vi "Arduino Interfacing VI.vi"(2 "error in (no error)":errorcluster, 3 "y Stepper value":u8, 4 "Data to Write":T1, 5 "AE Mode":T2) -> (0 "error out":errorcluster, 1 "Arduino Data":T3)   [LabVIEW 2018]
uses:
  Arduino_Interfacing.ctl
  I2C_MASTER_WRITE_NEW Type Def.ctl
  <vilib>/Studica/Studica Toolkit/Background/I2C Channel.ctl
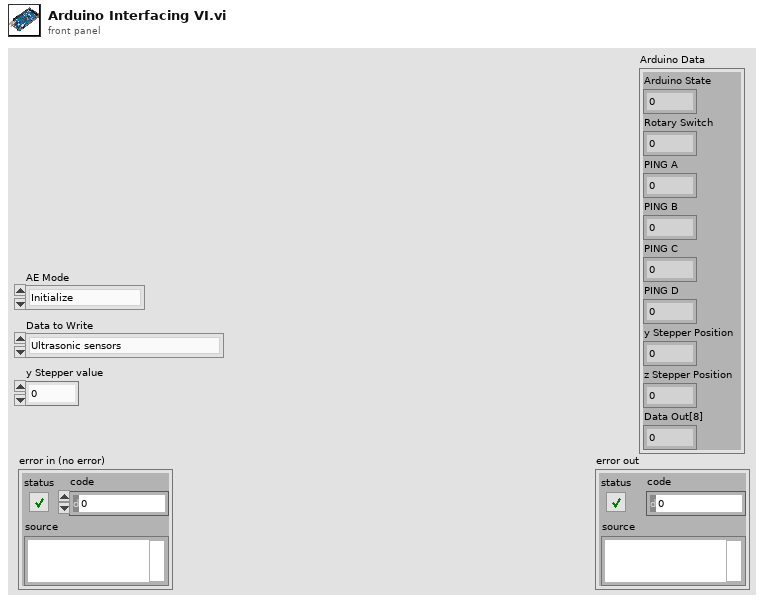
[diagram p1: front panel]
types:
  T1 = typedef "I2C_MASTER_WRITE_NEW Type Def.ctl" = enum16{"Ultrasonic sensors", "Stepper origin", "zStepper 13.3k", "zStepper 13k", "zStepper 12k", "zStepper 11k", "zStepper 10k", "zStepper 9k", "zStepper 8k", "zStepper 7k", "zStepper 6k", "zStepper 5k", "zStepper 4k", "zStepper 3k", "zStepper 2k", "zStepper 1k", "zStepper 900", "zStepper 800", "zStepper 700", "zStepper 600", "zStepper 500", "zStepper 400", "zStepper 300", "zStepper 200", "zStepper 100", "zStepper 0", "yStepper control", "Open Claw", "Close Claw", "Soft Reset"}
  T2 = typedef "Arduino_Interfacing.ctl" = enum16{"Initialize", "Write to Arduino", "Read From Arduino"}
  T3 = cluster{"Arduino State":u8, "Rotary Switch":u8, "PING A":u8, "PING B":u8, "PING C":u8, "PING D":u8, "y Stepper Position":u8, "z Stepper Position":u8, "Data Out[8]":u8}
  T4 = typedef "I2C Channel.ctl" = enum16{"Not Connected", "A", "B"}
  T5 = cluster{"I2C Channel":T4, "FPGA VI Reference Out":refnum<k20>}
  T6 = cluster{"Data Out[0]":u8, "Data Out[1]":u8, "Data Out[2]":u8, "Data Out[3]":u8, "Data Out[4]":u8, "Data Out[5]":u8, "Data Out[6]":u8, "Data Out[7]":u8, "Data Out[8]":u8}
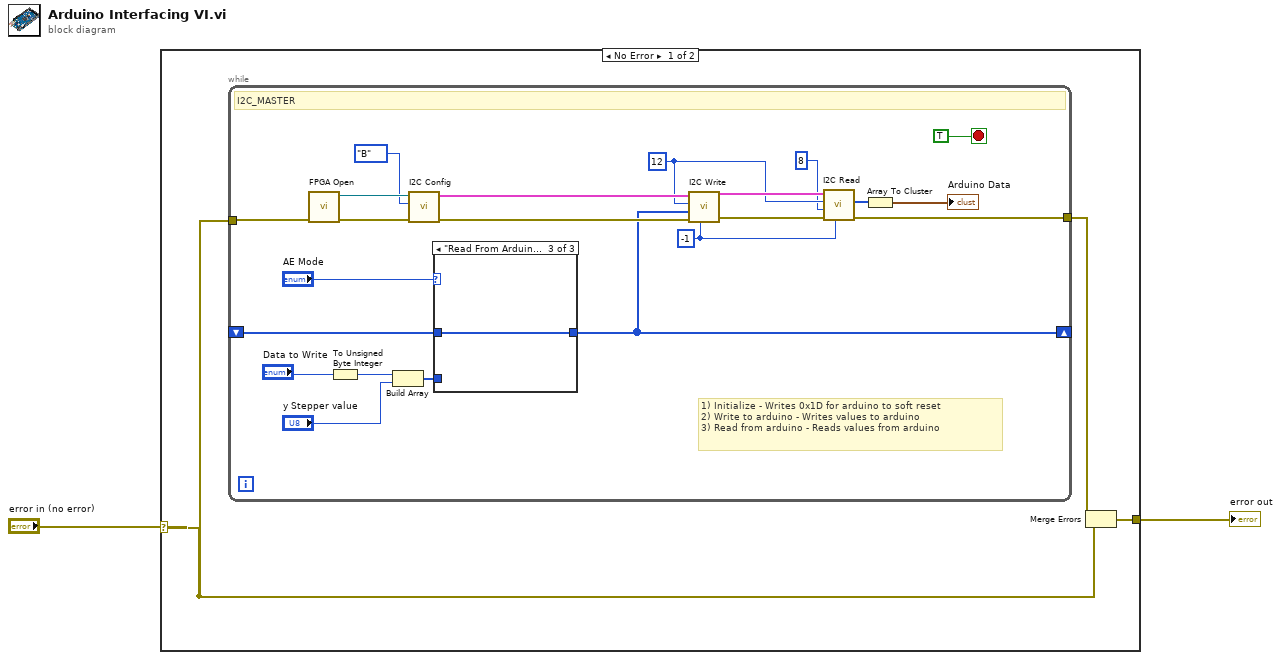
[diagram p0: block diagram]
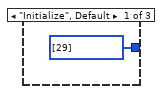
[diagram p2: hidden frame]
diagram:
  n1 = case shown="No Error" "error in (no error)" {
    selector: "error in (no error)" -> [w4 w31]
    tunnel: [w5 w31] -> w1
    frame No Error {
      n2 = while {
        tunnel: w4 -> [w21]
        shift-right: [w9] -> _
        shift-left: _ -> [w8]
        tunnel: [w13] -> w3
        stop <- TRUE ("stop") stop-if-true
        w16 = -1 ("Timeout ms (1000)")
        w15 = u8 12 ("Slave Address (7-bit)")
        # "1) Initialize - Writes 0x1D for arduino to soft reset\n2) Write to arduino - Writes values to arduino\n3) Read from arduino - Reads values from arduino"
        # "I2C_MASTER"
        n3 = call <vilib>:"FPGA Open.vi"("error in (no error)"=w21) -> ("error out"=w25:errorcluster, "FPGA Reference Out"=w26:refnum<k20>)  [unwired: 9 in]
        n4 = To Unsigned Byte Integer(number="Data to Write") -> (unsigned 8bit integer=w20:u8)
        n5 = Build Array(w20, "y Stepper value") -> (w10:u8[])
        n6 = call <vilib>:"I2C Config.vi"("error in (no error)"=w25, "I2C Channel"=I2C_Channel."B", "FPGA Reference"=w26) -> ("error out"=w22:errorcluster, "I2C Ref Out"=w23:T5)  [unwired: 7 in]
        n7 = case shown="\"Read From Arduino\"" "AE Mode" {
          tunnel: [u8[] [29] ("Data to Write") w29 w30] -> w9
          tunnel: w10 -> [_ w29 _]
          tunnel: w8 -> [_ _ w30]
          frame "Initialize", Default {
          }
          frame "Write to Arduino" {
          }
          frame "Read From Arduino" {
          }
        }
        n8 = call <vilib>:"I2C Write.vi"("Timeout ms (1000)"=w16, "error in (no error)"=w22, "Data to Write"=w9, "Slave Address (7-bit)"=w15, "I2C Ref In"=w23) -> ("error out"=w17:errorcluster, "I2C Ref Out"=w18:T5)  [unwired: 5 in]
        n9 = call <vilib>:"I2C Read.vi"("Timeout ms (1000)"=w16, "error in (no error)"=w17, "Bytes to Read"=u32 8, "Slave Address (7-bit)"=w15, "I2C Ref In"=w18) -> ("error out"=w13:errorcluster, "Data Out"=w12:u8[])  [unwired: 4 in, 1 out]
        n10 = Array To Cluster(array=w12) -> (cluster=→"Arduino Data":T6)
      }
      n11 = Merge Errors(w3, w4) -> (w5:errorcluster)
    }
    frame Error {
    }
  }
  "error out" <- w1
